vi "Set_CPP_BL.vi"(3 "Mode":T5, 5 "Traverse line In":T2 {"Carrier_2 Q (l/min)" format="%#.2f"; "Row Duration (mins)" format="%#.1f"; "Row No" min=0; "Trace Gas Concentration (%)" min=0.0 format="%#_4f"; "Carrier_1 Q (l/min)" format="%#.4f"; "Start X" format="%#.2f"; "Start Y" format="%#.2f"; "Start Z" format="%#.2f"; "End X" format="%#.2f"; "End Y" format="%#.2f"; "End Z" format="%#.2f"; "Tunnel Speed" format="%#.2f"; "Averaging time (mins)" min=0.0 format="%#.2f"}) -> (0 "Error Message":string, 1 "Status":T1, 2 "Traverse line Out":T2 {"Carrier_2 Q (l/min)" format="%#.2f"; "Row Duration (mins)" format="%#.1f"; "Row No" min=0; "Trace Gas Concentration (%)" min=0.0 format="%#_4f"; "Carrier_1 Q (l/min)" format="%#.4f"; "Start X" format="%#.2f"; "Start Y" format="%#.2f"; "Start Z" format="%#.2f"; "End X" format="%#.2f"; "End Y" format="%#.2f"; "End Z" format="%#.2f"; "Tunnel Speed" format="%#.2f"; "Averaging time (mins)" min=0.0 format="%#.2f"})   [LabVIEW 2021]
uses:
  Gen Trav/Multi_Run_Status.ctl
  CPPSW/Systems/Fetch/Fetch Sub VIs/NL_BL.ctl
  Gen Trav/Spacing.ctl
  Gen Trav/Traverse_cluster.ctl
  Controls/User_Specific_mode.ctl
  Controls/Multi_run_mode.ctl
panel:
  out "Rememberer":dbl[](array[numeric])
  out "Achieved Positions":dbl[](array[numeric])
  out "Requests (positive up from flush)":dbl[](array[numeric])
  # "Sets CPP's fetch/Boundary Layer based on inputs in the Comments box.\n\n• \"AllDown\" sets everything to zero; if Spires1 in use, they're set to 725 (their min)\n• \"Restore\" returns to the last non-zero setup.\n• \"LastBL-FILENAME\" sets everything to the last BL used in FILENAME.\n• \"NextBL-FILENAME\" sets everything to the next BL in FILENAME.\n• \"Specified-T1;T2;S1;S2;M1;M2;M3:B1;B2;B3\" sets the fetch to those explicit values."
  # "X           Y          Z"
  # "Start"
  # "End"
  # "X           Y          Z"
  # "Start"
  # "End"
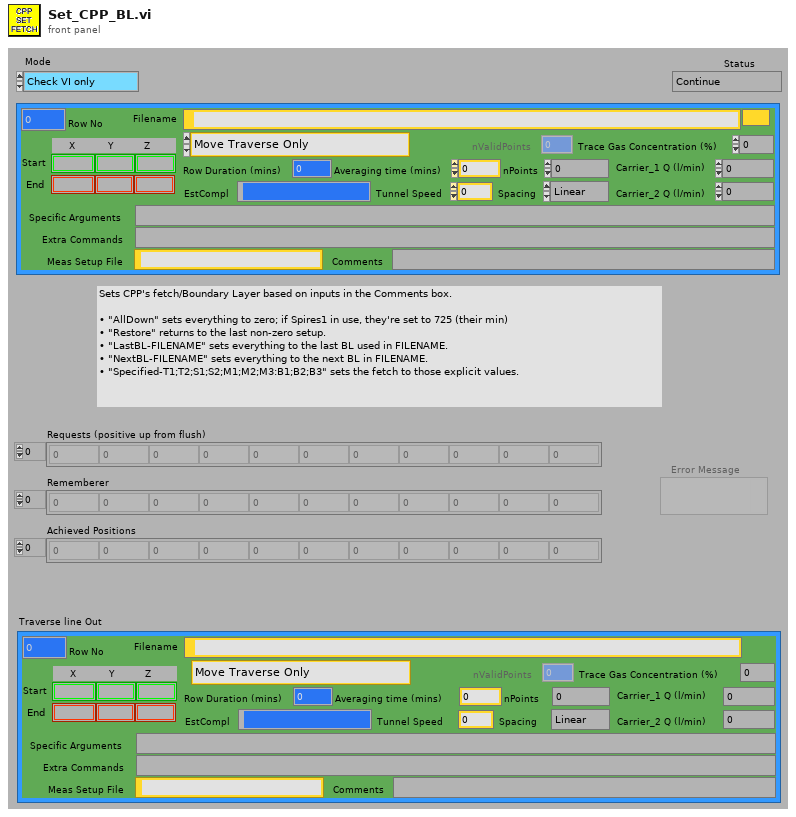
[diagram p1: front panel]
types:
  T1 = typedef "Multi_Run_Status.ctl" = enum16{"Continue", "Continue with Error", "Jump to Next Point", "Jump to Next Row", "Jump To Fall Back", "Terminate Run"}
  T2 = typedef "Traverse_cluster.ctl" = cluster{"Start X":sgl, "Start Y":sgl, "Start Z":sgl, "End X":sgl, "End Y":sgl, "End Z":sgl, "nPoints":i32, "Spacing":T3, "Filename":path, "Tunnel Speed":dbl, "Averaging time (mins)":dbl, "Extra Commands":string, "Carrier_1 Q (l/min)":dbl, "Carrier_2 Q (l/min)":dbl, "Trace Gas Concentration (%)":dbl, "Specific Arguments":string, "Comments":string, "Row No":i32, "Row Type Selector":T4, "EstCompl":string, "Row Duration (mins)":dbl, "nValidPoints":i32, "Meas Setup File":string}
  T3 = typedef "Spacing.ctl" = enum16{"Linear", "Log", "Gauss", "Specified", "N/A"}
  T4 = typedef "Multi_run_mode.ctl" = enum16{"Move Traverse Only", "Set Tunnel Speed Only", "Set Source Only", "Set Measurement Conditions", "Single Measurement", "Vertical Profile", "Lateral Profile", "Longitudinal Profile", "Multi-Axis Profile", "Explore Volume", "Auto Calibrate", "Meas Fast FID Bkgnd", "Check Beam Power", "Scanning Valve Measurement", "Run VI Named:", "Set ADAM Ch", "Wait (minutes)", "Send Message", "Synchronize With:", "Fall Back to this Row", "Turn Off Row Repeating", "Traverse 3D Volume", "Blank Row", "Jump to Fall Back Row"}
  T5 = typedef "User_Specific_mode.ctl" = enum16{"Check VI only", "Run VI"}
  T6 = typedef "NL_BL.ctl" = enum16{"Next", "Last"}
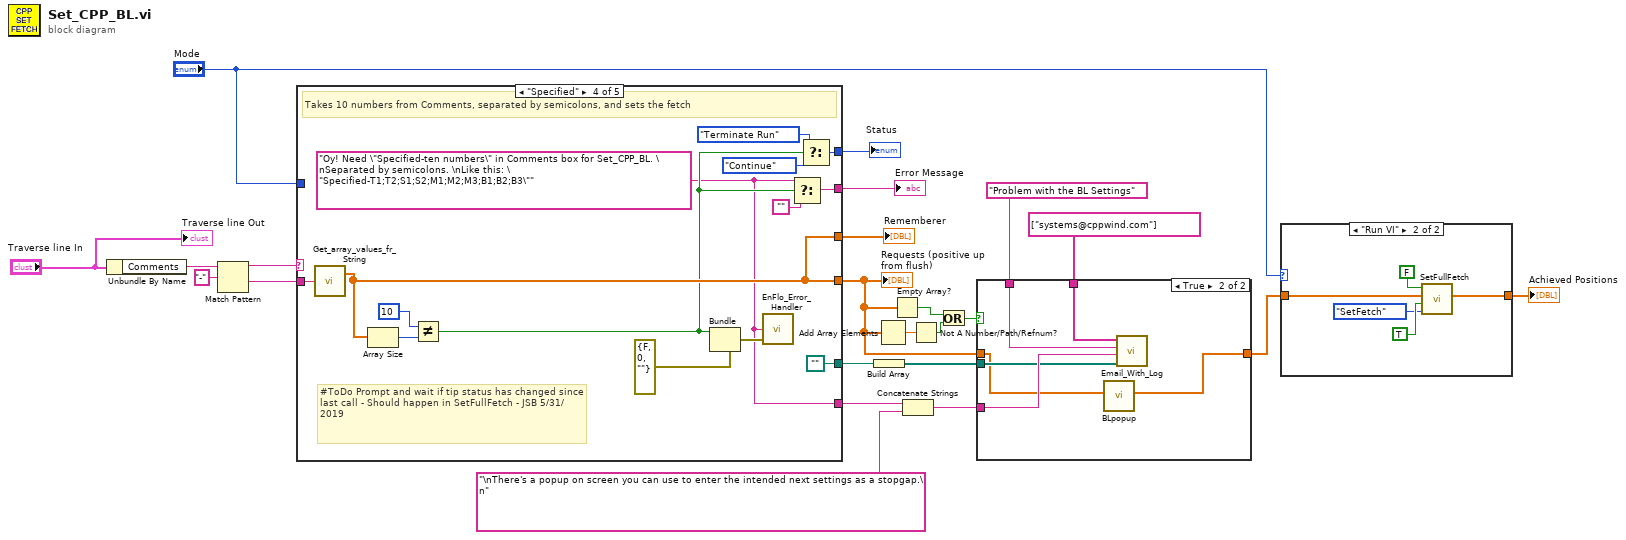
[diagram p0: block diagram]
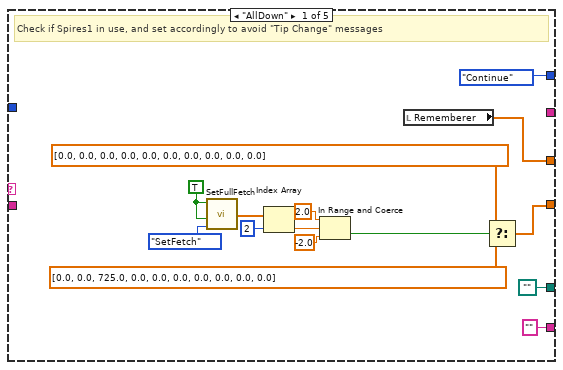
[diagram p4: hidden frame]
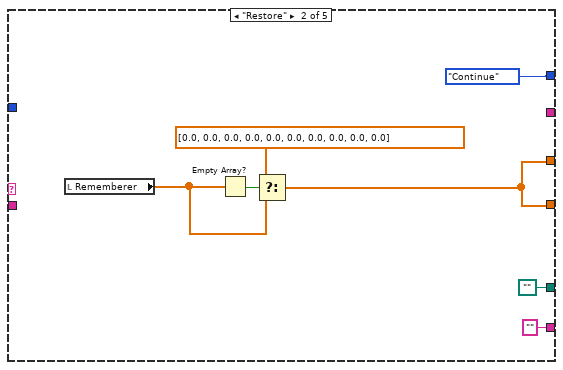
[diagram p5: hidden frame]
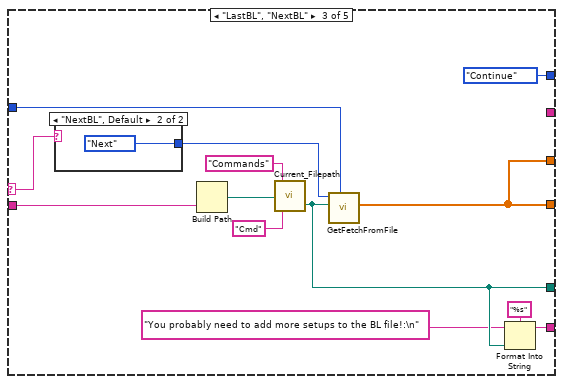
[diagram p6: hidden frame]
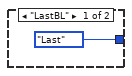
[diagram p7: hidden frame]
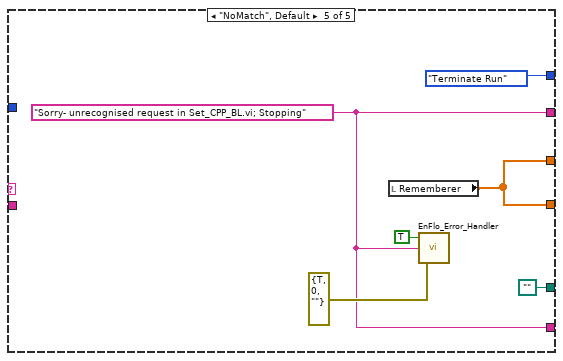
[diagram p8: hidden frame]
diagram:
  n1 = Unbundle By Name("Traverse line In") -> ("Comments"=w21:string)
  n2 = Match Pattern(string=w21, regular expression="-") -> (before substring=w20:string, after substring=w19:string)  [unwired: 1 in, 2 out]
  n3 = case shown="\"Specified\"" w20 {
    selector: w20 -> [_ _ w49 _ _]
    tunnel: [w27 w41 w52 w69 w80] -> w7
    tunnel: w19 -> [_ _ w55 w70 _]
    tunnel: [w38 w41 w52 w69 w80] -> w16
    tunnel: [Multi_Run_Status."Continue" ("Status") Multi_Run_Status."Continue" ("Status") Multi_Run_Status."Continue" ("Status") w68 Multi_Run_Status."Terminate Run" ("Status")] -> w18
    tunnel: [_ _ _ w65 w75] -> w15
    tunnel: [path "" ("Filename Out") path "" ("Filename Out") w50 path "" ("Filename Out") path "" ("Filename Out")] -> w4
    tunnel: "Mode" -> [_ _ w51 _ _]
    tunnel: ["" ("Error Type") "" ("Error Type") w46 w61 w75] -> w3
    frame "AllDown" {
      w34 = TRUE ("Mode")
      # "Check if Spires1 in use, and set accordingly to avoid \"Tip Change\" messages"
      n4 = call "SetFullFetch.vi"("Tab Control"=enum32{"SetFetch", "ZeroRampRoughness"}."SetFetch", "Multirun Control?"=w34, "Run Mode"=w34) -> ("Achieved Positions"=w33:dbl[])  [unwired: 8 in]
      n5 = Index Array(array=w33, index=2) -> (element=w31:dbl)
      n6 = In Range and Coerce(upper limit=2.0, x=w31, lower limit=-2.0) -> (In Range?=w26:bool)  [unwired: 1 out]
      n7 = local read "Rememberer"() -> (w38:dbl[])
      n8 = Select(t=dbl[] [0.0, 0.0, 0.0, 0.0, 0.0, 0.0, 0.0, 0.0, 0.0, 0.0] ("Requests (positive up from flush)"), s=w26, f=dbl[] [0.0, 0.0, 725.0, 0.0, 0.0, 0.0, 0.0, 0.0, 0.0, 0.0] ("Requests (positive up from flush)")) -> (s? t:f=w27:dbl[])
    }
    frame "Restore" {
      n9 = local read "Rememberer"() -> (w42:dbl[])
      n10 = Empty Array?(array=w42) -> (empty?=w43:bool)
      n11 = Select(t=dbl[] [0.0, 0.0, 0.0, 0.0, 0.0, 0.0, 0.0, 0.0, 0.0, 0.0] ("Achieved Positions"), s=w43, f=w42) -> (s? t:f=w41:dbl[])
    }
    frame "LastBL", "NextBL" {
      n12 = case shown="\"NextBL\", Default" w49 {
        tunnel: [NL_BL."Last" ("N/L BL") NL_BL."Next" ("N/L BL")] -> w54
        frame "LastBL" {
        }
        frame "NextBL", Default {
        }
      }
      n13 = Build Path(name or relative path=w55) -> (appended path=w56:path)  [unwired: 1 in]
      n14 = call "Current_Filepath.vi"("Short_Name"="Cmd", "Filename in"=w56, "Data Type"="Commands") -> ("Filename Out"=w50:path)  [unwired: 1 in, 1 out]
      n15 = call "GetFetchFromFile.vi"("Mode"=w51, "file path (dialog if empty)"=w50, "N/L BL"=w54) -> ("Current Requests"=w52:dbl[])  [unwired: 8 in]
      n16 = Format Into String(format string="%s", initial string="You probably need to add more setups to the BL file!:\n" ("message"), w50) -> (resulting string=w46:string)  [unwired: 1 in, 1 out]
    }
    frame "Specified" {
      w61 = "Oy! Need \"Specified-ten numbers\" in Comments box for Set_CPP_BL. \nSeparated by semicolons. \nLike this: \"Specified-T1;T2;S1;S2;M1;M2;M3;B1;B2;B3\"" ("message")
      # "#ToDo Prompt and wait if tip status has changed since last call - Should happen in SetFullFetch - JSB 5/31/2019"
      # "Takes 10 numbers from Comments, separated by semicolons, and sets the fetch"
      n17 = call "Get_array_values_fr_String.vi"("String Value"=w70) -> ("Numeric Array"=w69:dbl[])  [unwired: 1 out]
      n18 = Array Size(array=w69) -> (size(s)=w74:i32)
      n19 = Not Equal?(x=10, y=w74) -> (x != y?=w64:bool)
      n20 = Bundle(cluster=errorcluster {"status"=FALSE, "code"=0, "source"=""} ("error in (no error)"), "status"=w64) -> (w71:errorcluster)  [unwired: 2 in]
      n21 = call "EnFlo_Error_Handler.vi"("error in (no error)"=w71, "Error Type"=w61) -> ()  [unwired: 2 in, 2 out]
      n22 = Select(t=w61, s=w64, f="") -> (s? t:f=w65:string)
      n23 = Select(t=Multi_Run_Status."Terminate Run" ("Status"), s=w64, f=Multi_Run_Status."Continue" ("Status")) -> (s? t:f=w68:T1)
    }
    frame "NoMatch", Default {
      w75 = "Sorry- unrecognised request in Set_CPP_BL.vi; Stopping" ("Error Type")
      n24 = local read "Rememberer"() -> (w80:dbl[])
      n25 = call "EnFlo_Error_Handler.vi"("error in (no error)"=errorcluster {"status"=TRUE, "code"=0, "source"=""}, "Error Type"=w75, "Dialog Box (F)"=TRUE ("Dialog Box (T)")) -> ()  [unwired: 1 in, 2 out]
    }
  }
  "Error Message" <- w15
  "Status" <- w18
  "Requests (positive up from flush)" <- w7
  "Rememberer" <- w16
  n26 = Build Array(w4) -> (w9:path[])
  n27 = Add Array Elements(numeric array=w7) -> (sum=w13:dbl)
  n28 = Empty Array?(array=w7) -> (empty?=w5:bool)
  n29 = Concatenate Strings(w3, "\nThere's a popup on screen you can use to enter the intended next settings as a stopgap.\n" ("message")) -> (w2:string)
  n30 = Not A Number/Path/Refnum?(number/path/refnum=w13) -> (NaN/Path/Refnum?=w14:bool)
  n31 = Or(x=w5, y=w14) -> (x .or. y?=w6:bool)
  n32 = case shown="True" w6 {
    tunnel: [w81 w83] -> w12
    tunnel: w7 -> [w81 w82]
    tunnel: string[] ["systems@cppwind.com"] ("recipients") -> [_ w87]
    tunnel: "Problem with the BL Settings" -> [_ w86]
    tunnel: w2 -> [_ w85]
    tunnel: w9 -> [_ w84]
    frame False {
    }
    frame True {
      n33 = call "BLpopup.vi"("deliveredBLarray"=w82) -> ("emergencyBLarray"=w83:dbl[])  [unwired: 10 in]
      n34 = call "Email_With_Log.vi"("recipients"=w87, "subject ([No Subject])"=w86, "message"=w85, "attachments"=w84) -> ()  [unwired: 1 in, 2 out]
    }
  }
  n35 = case shown="\"Run VI\"" "Mode" {
    tunnel: [w88 w92] -> w17
    tunnel: w12 -> [w88 w91]
    frame "Check VI only", Default {
    }
    frame "Run VI" {
      n36 = call "SetFullFetch.vi"("Tab Control"=enum32{"SetFetch", "ZeroRampRoughness"}."SetFetch", "Multirun Control?"=TRUE, "DemandsFromAbove"=w91, "Run Mode"=FALSE ("Mode")) -> ("Achieved Positions"=w92:dbl[])  [unwired: 7 in]
    }
  }
  "Achieved Positions" <- w17
  "Traverse line Out" <- "Traverse line In"
